vi "control-node.vi"() -> ()   [LabVIEW 2024]
panel:
  out "error out":errorcluster
  out "Reader URL":string
  out "Waveform Chart":dbl[][](graph)
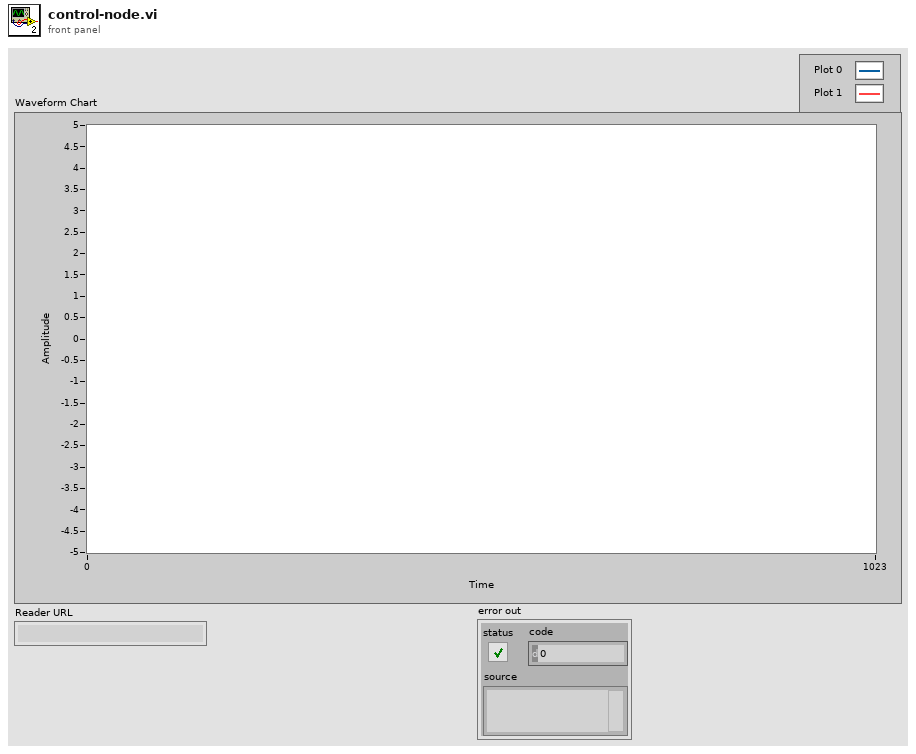
[diagram p1: front panel]
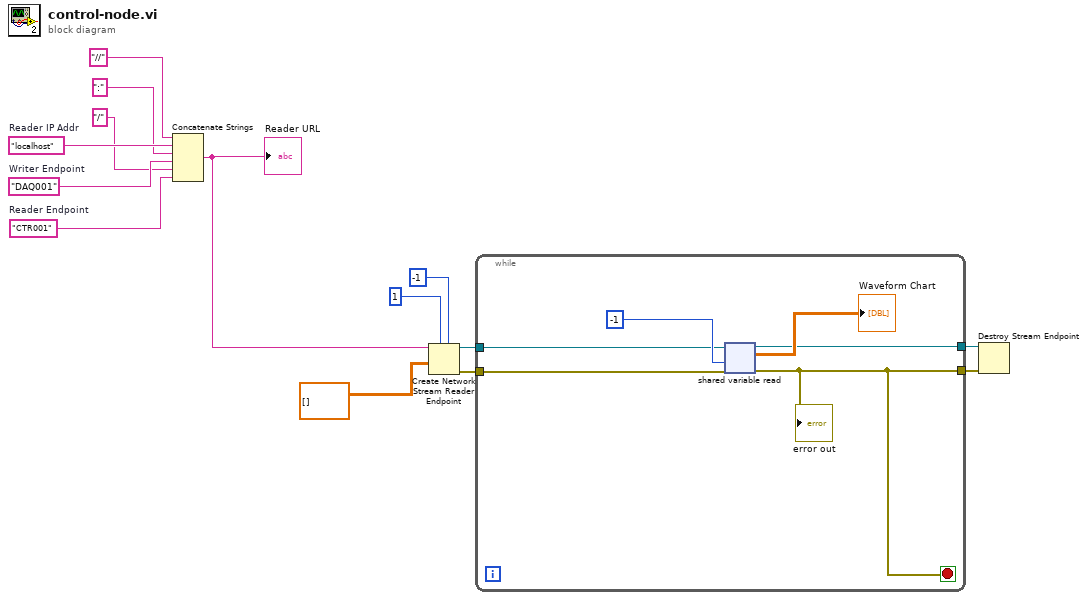
[diagram p0: block diagram]
diagram:
  w11 = "DAQ001"  # Writer Endpoint
  w13 = "localhost"  # Reader IP Addr
  w9 = "CTR001"  # Reader Endpoint
  n1 = Concatenate Strings("//" ("string"), w13, ":" ("string"), w11, "/" ("string"), w9) -> (w1:string)
  "Reader URL" <- w1
  n2 = Create Network Stream Reader Endpoint(5:-1 ("timeout in ms (-1)"), 7:1 ("writer buffer size"), 9:dbl[][] [], 11:w1) -> (0:w8:errorcluster, 3:w6:refnum<k21>)  [unwired: 3 in]
  n3 = while {
    tunnel: w8 -> [w18]
    tunnel: w6 -> [w17]
    tunnel: [w16] -> w5
    tunnel: [w15] -> w4
    stop <- w15 stop-if-true
    n4 = shared-variable-read(w17, w18, -1 ("timeout ms (-1)")) -> (w16:refnum<k21>, w15:errorcluster, →"Waveform Chart":dbl[][])  [unwired: 1 out]
    "error out" <- w15
  }
  n5 = Destroy Stream Endpoint(8:w4, 11:w5) -> ()  [unwired: 1 out]
